vi "Write Payload.vi"(10 "Payload":string, 11 "GDSII.DataType.Word in":refnum<class "GDSII.DataType.Word.lvclass">) -> (3 "GDSII.DataType.Word out":refnum<class "GDSII.DataType.Word.lvclass">)   [LabVIEW 2019, in "GDSII.DataType.Word.lvclass"]
uses:
  GDSII.DataType.Word.lvclass
  GDSII.DataType.Word.lvclass/GDSII.DataType.Word.ctl
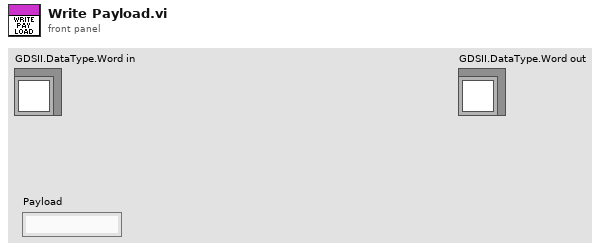
[diagram p1: front panel]
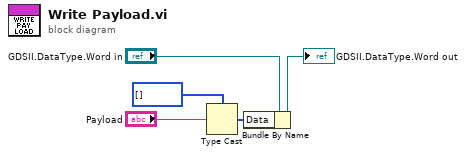
[diagram p0: block diagram]
diagram:
  n1 = Type Cast(type=i16[] [], x="Payload") -> (*(type *) &x=w3:i16[])
  n2 = Bundle By Name(cluster="GDSII.DataType.Word in", "Data"=w3) -> (→"GDSII.DataType.Word out":refnum<class "GDSII.DataType.Word.lvclass">)
